vi "CheckPassFailOutputs.vi"(8 "error in":errorcluster, 10 "test vi reference":refnum<vi>, 11 "TestCase in":refnum<class "TestCase.lvclass">) -> (0 "error out":errorcluster, 3 "TestCase out":refnum<class "TestCase.lvclass">)   [LabVIEW 2011, in "TestCase.lvclass"]
doc: "Checks for Pass and Fail indicators. If either or both is found then check their status to determine if test passed or failed."
uses:
  TestCase.lvclass
  Libraries/VITesterUtilities.lvlib
panel:
  # "JKI VI Tester for LabVIEW\nhttp://jkisoft.com/vi-tester\nCopyright (C) 2007-2009, JKI <info@jkisoft.com>\nALL RIGHTS RESERVED"
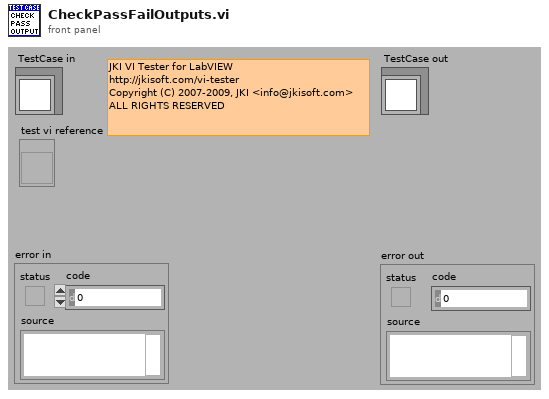
[diagram p1: front panel]
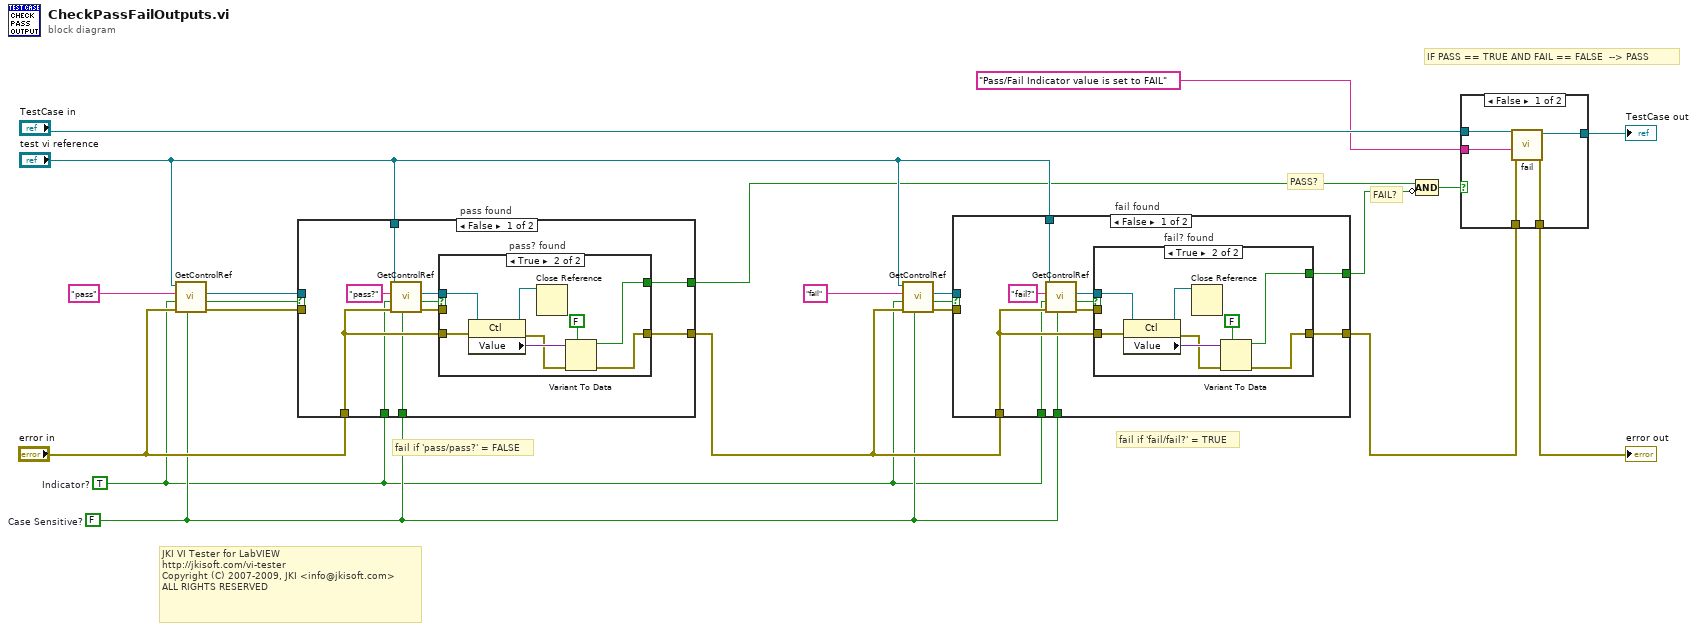
[diagram p0: block diagram]
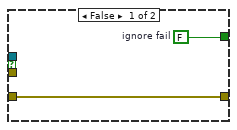
[diagram p3: hidden frame]
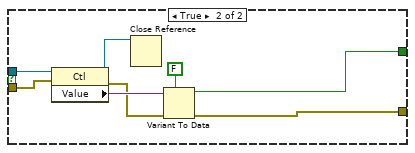
[diagram p4: hidden frame]
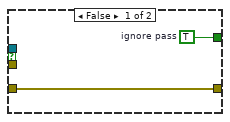
[diagram p5: hidden frame]
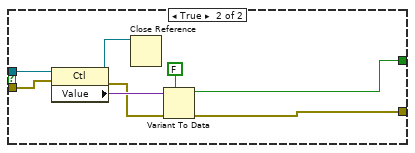
[diagram p6: hidden frame]
diagram:
  w2 = FALSE  # Case Sensitive?
  w1 = TRUE  # Indicator?
  # "JKI VI Tester for LabVIEW\nhttp://jkisoft.com/vi-tester\nCopyright (C) 2007-2009, JKI <info@jkisoft.com>\nALL RIGHTS RESERVED"
  # "FAIL?"
  # "PASS?"
  # "IF PASS == TRUE AND FAIL == FALSE  --> PASS"
  # "fail if 'pass/pass?' = FALSE"
  # "fail if 'fail/fail?' = TRUE"
  n1 = call "GetControlRef.vi"("Case Sensitive? (TRUE)"=w2, "error in (no error)"="error in", "Indicator (F=Control)"=w1, "Control Name"="pass", "VI Refnum"="test vi reference") -> ("error out"=w15:errorcluster, "Found?"=w17:bool, "Ctl Refnum"=w16:refnum<vi>)  [unwired: 4 in]
  n2 = case "pass found" shown="False" w17 {
    tunnel: "test vi reference" -> [w30 _]
    tunnel: "error in" -> [w26 _]
    tunnel: w16 -> [_ w49]
    tunnel: w15 -> [_ w45]
    tunnel: [w27 w44] -> w9
    tunnel: [w24 w42] -> w5
    tunnel: w2 -> [w23 _]
    tunnel: w1 -> [w22 _]
    frame False {
      n3 = call "GetControlRef.vi"("Case Sensitive? (TRUE)"=w23, "error in (no error)"=w26, "Indicator (F=Control)"=w22, "Control Name"="pass?", "VI Refnum"=w30) -> ("error out"=w28:errorcluster, "Found?"=w29:bool, "Ctl Refnum"=w25:refnum<vi>)  [unwired: 4 in]
      n4 = case "pass? found" shown="True" w29 {
        tunnel: w28 -> [_ _]
        tunnel: [w33 w37] -> w27
        tunnel: w26 -> [w33 w38]
        tunnel: w25 -> [_ w35]
        tunnel: [w32 w34] -> w24
        frame False {
          w32 = TRUE  # ignore pass
        }
        frame True {
          n5 = property class="Ctl"(reference=w35, error in=w38) -> (reference out=w36:refnum<vi>, error out=w39:errorcluster, "Value"=w41:variant)
          n6 = Close Reference(reference=w36) -> ()  [unwired: 1 in, 1 out]
          n7 = Variant To Data(error in=w39, type=FALSE, Variant=w41) -> (data=w34:bool, error out=w37:errorcluster)
        }
      }
    }
    frame True {
      n8 = property class="Ctl"(reference=w49, error in=w45) -> (reference out=w43:refnum<vi>, error out=w46:errorcluster, "Value"=w48:variant)
      n9 = Close Reference(reference=w43) -> ()  [unwired: 1 in, 1 out]
      n10 = Variant To Data(error in=w46, type=FALSE, Variant=w48) -> (data=w42:bool, error out=w44:errorcluster)
    }
  }
  n11 = call "GetControlRef.vi"("Case Sensitive? (TRUE)"=w2, "error in (no error)"=w9, "Indicator (F=Control)"=w1, "Control Name"="fail", "VI Refnum"="test vi reference") -> ("error out"=w13:errorcluster, "Found?"=w11:bool, "Ctl Refnum"=w12:refnum<vi>)  [unwired: 4 in]
  n12 = case "fail found" shown="False" w11 {
    tunnel: "test vi reference" -> [w58 _]
    tunnel: w9 -> [w54 _]
    tunnel: w12 -> [_ w77]
    tunnel: w13 -> [_ w73]
    tunnel: [w55 w72] -> w8
    tunnel: [w52 w70] -> w6
    tunnel: w2 -> [w51 _]
    tunnel: w1 -> [w50 _]
    frame False {
      n13 = call "GetControlRef.vi"("Case Sensitive? (TRUE)"=w51, "error in (no error)"=w54, "Indicator (F=Control)"=w50, "Control Name"="fail?", "VI Refnum"=w58) -> ("error out"=w56:errorcluster, "Found?"=w57:bool, "Ctl Refnum"=w53:refnum<vi>)  [unwired: 4 in]
      n14 = case "fail? found" shown="True" w57 {
        tunnel: w56 -> [_ _]
        tunnel: [w61 w65] -> w55
        tunnel: w54 -> [w61 w66]
        tunnel: w53 -> [_ w63]
        tunnel: [w60 w62] -> w52
        frame False {
          w60 = FALSE  # ignore fail
        }
        frame True {
          n15 = property class="Ctl"(reference=w63, error in=w66) -> (reference out=w64:refnum<vi>, error out=w67:errorcluster, "Value"=w69:variant)
          n16 = Close Reference(reference=w64) -> ()  [unwired: 1 in, 1 out]
          n17 = Variant To Data(error in=w67, type=FALSE, Variant=w69) -> (data=w62:bool, error out=w65:errorcluster)
        }
      }
    }
    frame True {
      n18 = property class="Ctl"(reference=w77, error in=w73) -> (reference out=w71:refnum<vi>, error out=w74:errorcluster, "Value"=w76:variant)
      n19 = Close Reference(reference=w71) -> ()  [unwired: 1 in, 1 out]
      n20 = Variant To Data(error in=w74, type=FALSE, Variant=w76) -> (data=w70:bool, error out=w72:errorcluster)
    }
  }
  n21 = Compound Arithmetic op=AND(w5, invert w6) -> (w4:bool)
  n22 = case shown="False" w4 {
    tunnel: [w82 w84] -> w21
    tunnel: "TestCase in" -> [w81 w84]
    tunnel: [w80 w83] -> w19
    tunnel: w8 -> [w79 w83]
    tunnel: "Pass/Fail Indicator value is set to FAIL" ("Control Name") -> [w78 _]
    frame False {
      n23 = call-dynamic "fail.vi"("error in (no error)"=w79, "message (\"\")"=w78, "TestCase in"=w81) -> ("error out"=w80:errorcluster, "TestCase out"=w82:refnum<class "TestCase.lvclass">)  [unwired: 7 in]
    }
    frame True {
      # "pass"
    }
  }
  "TestCase out" <- w21
  "error out" <- w19
